vi "WheelShooter Open.vi"(1 "error in":errorcluster, 2 "input cluster":T2) -> (0 "error out":errorcluster)   [LabVIEW 2015]
doc: "Opens refnums to two motors and a servo(connected via Talon SRX without CAN) for a dual flywheel ball shooter. If the motors are arranged vertically, B is the bottom one."
uses:
  <vilib>/Rock Robotics/WPI/Solenoid/WPI_SolenoidChannel.ctl
  <vilib>/Rock Robotics/WPI/CAN/TalonSRX/WPI_CANTalonSRX_APIControlMode.ctl
  <vilib>/Rock Robotics/WPI/SafetyOutput/WPI_SafetyOutputConfigMenu.ctl
  <vilib>/Rock Robotics/WPI/Solenoid/WPI_SolenoidOpenSingle.vi
  <vilib>/Rock Robotics/WPI/MotorControl/WPI_MotorControlOpenCANTalonSRX.vi
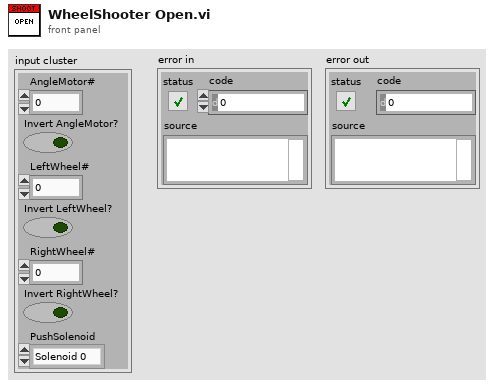
[diagram p1: front panel]
types:
  T1 = typedef "WPI_SolenoidChannel.ctl" = enum8{"Solenoid 0", "Solenoid 1", "Solenoid 2", "Solenoid 3", "Solenoid 4", "Solenoid 5", "Solenoid 6", "Solenoid 7", "Invalid"}
  T2 = cluster{"AngleMotor#":u8, "Invert AngleMotor?":bool, "LeftWheel#":u8, "Invert LeftWheel?":bool, "RightWheel#":u8, "Invert RightWheel?":bool, "PushSolenoid":T1}
  T3 = typedef "WPI_SafetyOutputConfigMenu.ctl" = enum16{"Enable", "Disable"}
  T4 = typedef "WPI_CANTalonSRX_APIControlMode.ctl" = enum8{"Percent VBus", "Speed", "Position", "Slave", "Unchanged / Invalid", "Voltage Compensation", "Current", "Motion Profile"}
  T5 = typedef "WPI_MotorControlDeviceRef.ctl" = cluster{"DeviceStatus":errorcluster, "Type":T6, "PWM":cluster{"PWM Channel":T7, "DeadBand":T8}, "CAN":cluster{"Device Number":u8, "Control Mode":T9, "Semaphore":T10, "Max Vout":dbl, "TalonSRX Control Mode":T4}, "Invert":bool}
  T6 = typedef "WPI_MotorControlType.ctl" = enum16{"PWM", "CAN", "CANTalonSRX"}
  T7 = typedef "FPGA_DIOPWMChannel.ctl" = enum8{"PWM 0", "PWM 1", "PWM 2", "PWM 3", "PWM 4", "PWM 5", "PWM 6", "PWM 7", "PWM 8", "PWM 9", "PWM MXP 0", "PWM MXP 1", "PWM MXP 2", "PWM MXP 3", "PWM MXP 4", "PWM MXP 5", "PWM MXP 6", "PWM MXP 7", "PWM MXP 8", "PWM MXP 9", "Invalid"}
  T8 = typedef "WPI_PWMDeadband.ctl" = cluster{"Name":string, "maxPositivePwm":i32, "minPositivePwm":i32, "centerPwm":i32, "maxNegativePwm":i32, "minNegativePwm":i32, "angularRange":u16}
  T9 = typedef "WPI_CANJaguar_ControlMode.ctl" = enum8{"Percent VBus", "Current", "Speed", "Position", "Voltage"}
  T10 = typedef "Semaphore RefNum" = refnum<k1>
  T11 = typedef "WPI_SolenoidDevRef.ctl" = cluster{"DevStatus":errorcluster, "Pneumatics Control Module":u8, "Forward Solenoid Channel":T1, "Reverse Solenoid Channel":T1}
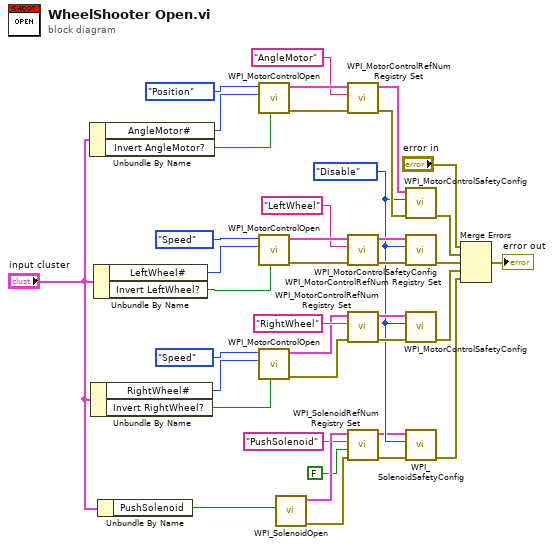
[diagram p0: block diagram]
diagram:
  w2 = WPI_SafetyOutputConfigMenu."Disable" ("mode")
  n1 = Unbundle By Name("input cluster") -> ("AngleMotor#"=w16:u8, "Invert AngleMotor?"=w15:bool)
  n2 = Unbundle By Name("input cluster") -> ("RightWheel#"=w12:u8, "Invert RightWheel?"=w11:bool)
  n3 = Unbundle By Name("input cluster") -> ("LeftWheel#"=w14:u8, "Invert LeftWheel?"=w13:bool)
  n4 = Unbundle By Name("input cluster") -> ("PushSolenoid"=w6:T1)
  n5 = call-poly <vilib>:"WPI_MotorControlOpen.vi"("Invert"=w15, "Device Number"=w16, "Control Mode"=WPI_CANTalonSRX_APIControlMode."Position") -> ("error out"=w39:errorcluster, "MotorControlDeviceRef"=w38:T5)  [unwired: 7 in]
  n6 = call-poly <vilib>:"WPI_MotorControlOpen.vi"("Invert"=w13, "Device Number"=w14, "Control Mode"=WPI_CANTalonSRX_APIControlMode."Speed") -> ("error out"=w37:errorcluster, "MotorControlDeviceRef"=w36:T5)  [unwired: 7 in]
  n7 = call-poly <vilib>:"WPI_MotorControlOpen.vi"("Invert"=w11, "Device Number"=w12, "Control Mode"=WPI_CANTalonSRX_APIControlMode."Speed") -> ("error out"=w26:errorcluster, "MotorControlDeviceRef"=w28:T5)  [unwired: 7 in]
  n8 = call-poly <vilib>:"WPI_SolenoidOpen.vi"("Solenoid Channel"=w6) -> ("error out"=w9:errorcluster, "SolenoidDevRef"=w10:T11)  [unwired: 9 in]
  n9 = call <vilib>:"WPI_MotorControlRefNum Registry Set.vi"("error in (no error)"=w39, "refnum name"="AngleMotor", "MotorControlDevRef"=w38) -> ("error out"=w23:errorcluster, "MotorControlDevRef"=w17:T5)  [unwired: 7 in]
  n10 = call <vilib>:"WPI_MotorControlRefNum Registry Set.vi"("error in (no error)"=w37, "refnum name"="LeftWheel", "MotorControlDevRef"=w36) -> ("error out"=w21:errorcluster, "MotorControlDevRef"=w18:T5)  [unwired: 7 in]
  n11 = call <vilib>:"WPI_MotorControlRefNum Registry Set.vi"("error in (no error)"=w26, "refnum name"="RightWheel", "MotorControlDevRef"=w28) -> ("error out"=w25:errorcluster, "MotorControlDevRef"=w24:T5)  [unwired: 7 in]
  n12 = call <vilib>:"WPI_SolenoidRefNum Registry Set.vi"("error in (no error)"=w9, "Test Mode Only"=FALSE, "refnum name"="PushSolenoid", "SolenoidDevRef"=w10) -> ("error out"=w3:errorcluster, "SolenoidDevRef"=w1:T11)  [unwired: 6 in]
  n13 = call <vilib>:"WPI_MotorControlSafetyConfig.vi"("error in (no error)"=w23, "mode"=w2, "MotorControlDevRef"=w17) -> ("error out"=w22:errorcluster)  [unwired: 7 in, 1 out]
  n14 = call <vilib>:"WPI_MotorControlSafetyConfig.vi"("error in (no error)"=w21, "mode"=w2, "MotorControlDevRef"=w18) -> ("error out"=w20:errorcluster)  [unwired: 7 in, 1 out]
  n15 = call <vilib>:"WPI_MotorControlSafetyConfig.vi"("error in (no error)"=w25, "mode"=w2, "MotorControlDevRef"=w24) -> ("error out"=w19:errorcluster)  [unwired: 7 in, 1 out]
  n16 = call <vilib>:"WPI_SolenoidSafetyConfig.vi"("error in (no error)"=w3, "mode"=w2, "SolenoidDevRef"=w1) -> ("error out"=w4:errorcluster)  [unwired: 7 in, 1 out]
  n17 = Merge Errors("error in", w22, w20, w19, w4) -> (→"error out":errorcluster)
